vi "Sound_gen2.vi"(6 "Sound time(s)":dbl=1.0, 7 "Dit time(ms)":u32, 8 "stop":bool, 9 "Sound On/Off":bool=TRUE, 10 "Frequency":dbl, 11 "Volume":dbl(knob) scale=0.0..100.0) -> (0 "error out":errorcluster)   [LabVIEW 2022 SP3]
uses:
  <vilib>/sound2/lvsound2.llb/Sound Data Format.ctl
  <vilib>/sound2/lvsound2.llb/Sampling Mode.ctl
  <vilib>/sound2/lvsound2.llb/Sound Output Set Volume (Single).vi
  <vilib>/sound2/lvsound2.llb/Sound Output Write (DBL Single).vi
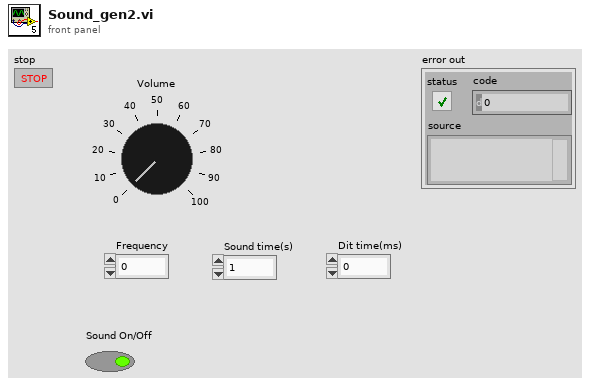
[diagram p1: front panel]
types:
  T1 = typedef "Sampling Mode.ctl" = i32
  T2 = typedef "Sound Data Format.ctl" = cluster{"sample rate (S/s)":dbl, "number of channels":i32, "bits per sample":i32}
  T3 = typedef "Sound Output Task ID.ctl" = u32
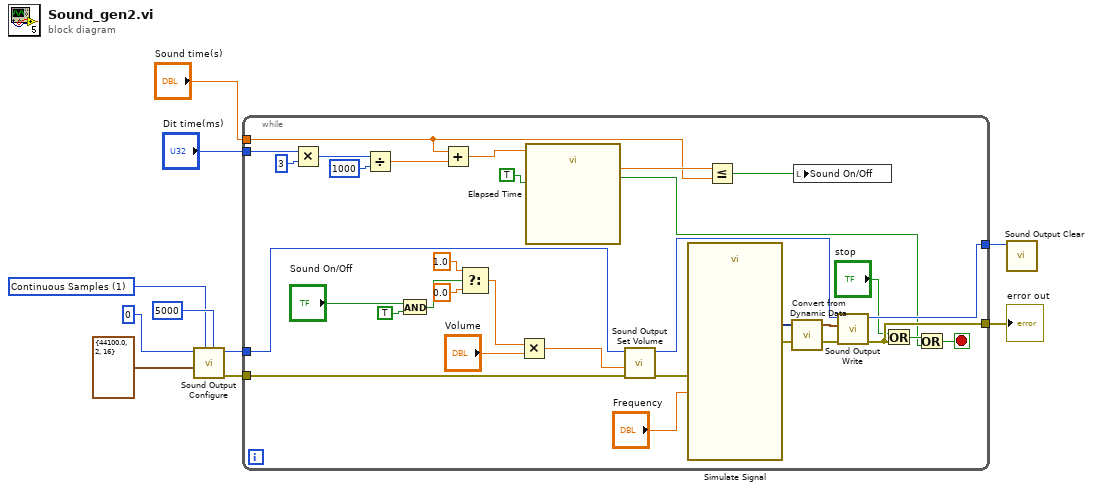
[diagram p0: block diagram]
diagram:
  w7 = T1 1 items=["Finite Samples", "Continuous Samples"] ("sample mode")
  n1 = call <vilib>:"Sound Output Configure.vi"("number of samples/ch"=5000, "sample mode"=w7, "sound format"=T2 {"sample rate (S/s)"=44100.0, "number of channels"=2, "bits per sample"=16}, "device ID"=u32 0) -> ("error out"=w5:errorcluster, "task ID"=w6:T3)  [unwired: 6 in]
  n2 = while {
    tunnel: w6 -> [w42]
    tunnel: [w39] -> w3
    tunnel: w5 -> [w41]
    tunnel: [w40] -> w4
    tunnel: "Sound time(s)" -> [w11]
    tunnel: "Dit time(ms)" -> [w20]
    stop <- w21 stop-if-true
    n3 = Multiply(x=w20, y=u32 3) -> (x*y=w14:u32)
    n4 = Divide(x=w14, y=u32 1000 ("x")) -> (x/y=w12:dbl)
    n5 = And(x="Sound On/Off", y=TRUE) -> (x .and. y?=w30:bool)
    n6 = Add(x=w11, y=w12) -> (x+y=w17:dbl)
    n7 = Select(t=1.0, s=w30, f=0.0) -> (s? t:f=w26:dbl)
    n8 = Multiply(x=w26, y="Volume") -> (x*y=w25:dbl)
    n9 = call "Elapsed Time"("Time Target (s)"=w17, "Auto Reset"=TRUE) -> ("Elapsed Time (s)"=w16:dbl, "Time has Elapsed"=w18:bool)  [unwired: 10 in, 6 out]
    n10 = call-poly <vilib>:"Sound Output Set Volume.vi"("error in (no error)"=w41, "volume"=w25, "task ID"=w42) -> ("error out"=w37:errorcluster, "task ID out"=w35:T3)  [unwired: 7 in]
    n11 = call "Simulate Signal"("Frequency"="Frequency", "error in (no error)"=w37) -> ("Sine"=w36:dynamicdata, "error out"=w33:errorcluster)  [unwired: 12 in]
    n12 = Less Or Equal?(x=w16, y=w11) -> (x <= y?=w15:bool)
    n13 = call "Convert from Dynamic Data"("Dynamic Data Type"=w36) -> ("Waveform"=w34:waveform(dbl))  [unwired: 3 in]
    n14 = local write "Sound On/Off"(w15) -> ()
    n15 = call-poly <vilib>:"Sound Output Write.vi"("error in (no error)"=w33, "data"=w34, "task ID"=w35) -> ("error out"=w40:errorcluster, "task ID out"=w39:T3)  [unwired: 7 in]
    n16 = Or(x="stop", y=w40) -> (x .or. y?=w22:bool)
    n17 = Or(x=w22, y=w18) -> (x .or. y?=w21:bool)
  }
  "error out" <- w4
  n18 = call <vilib>:"Sound Output Clear.vi"("task ID"=w3) -> ()  [unwired: 10 in, 1 out]
